vi "SaveParameterFile.vi"(8 "error in (no error)":errorcluster, 9 "Parameter File path and name":path, 11 "controller in":refnum<k24>) -> (0 "error out":errorcluster, 2 "Error Status":bool, 3 "controller out":refnum<k24>)   [LabVIEW 2021]
uses:
  C:/Program Files (x86)/Aerotech/A3200/LabVIEW/2010/Bin/Aerotech.A3200.dll
  Bin/Aerotech.A3200.dll
  C:/Program Files (x86)/Aerotech/A3200/LabVIEW/2010/Bin/Aerotech.A3200.LabVIEW.dll
  Bin/Aerotech.A3200.LabVIEW.dll
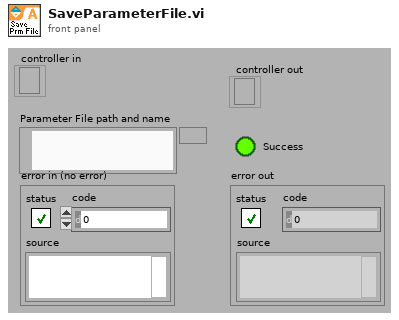
[diagram p1: front panel]
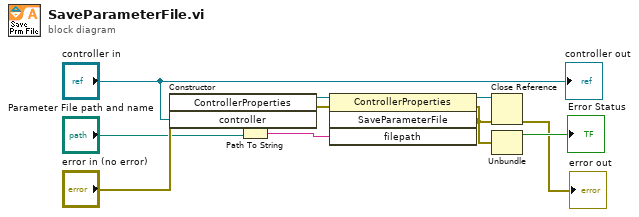
[diagram p0: block diagram]
diagram:
  n1 = constructor class="ControllerProperties"(error in="error in (no error)", "controller"="controller in") -> (reference out=w5:refnum<k24>, error out=w4:errorcluster)  [unwired: 2 in, 2 out]
  n2 = Path To String(path="Parameter File path and name") -> (string=w2:string)
  n3 = invoke class="ControllerProperties" method="SaveParameterFile"(reference=w5, error in=w4, "filepath"=w2) -> (reference out=w3:refnum<k24>, error out=w1:errorcluster)  [unwired: 1 in, 2 out]
  n4 = Close Reference(reference=w3, error in (no error)=w1) -> (error out=→"error out":errorcluster)
  n5 = Unbundle(w1) -> ("status"=→"Error Status":bool)  [unwired: 2 out]
  "controller out" <- "controller in"
